vi "Power Supply Loop.vi"(11 "FPGA Ref":T1) -> ()   [LabVIEW 2013]
uses:
  Controls/FPGA_Reference.ctl
  <vilib>/rvi/interface/nirviReadWriteControl/nirviReadWriteControl.xnode
  FPGA Bitfiles/LSDurability_Main.lvbitx
  <vilib>/rvi/errors/niLvFpgaMergeErrorWithErrorCode.vi
  <vilib>/rvi/errors/niLvFpgaAdjustHostInterfaceError.vi
panel:
  in  "Power Supply Cmd (V):":dbl min=0.0 max=20.0 format="%#.2f"
  in  "Closed Loop Voltage":bool
  out "FreezePID":bool
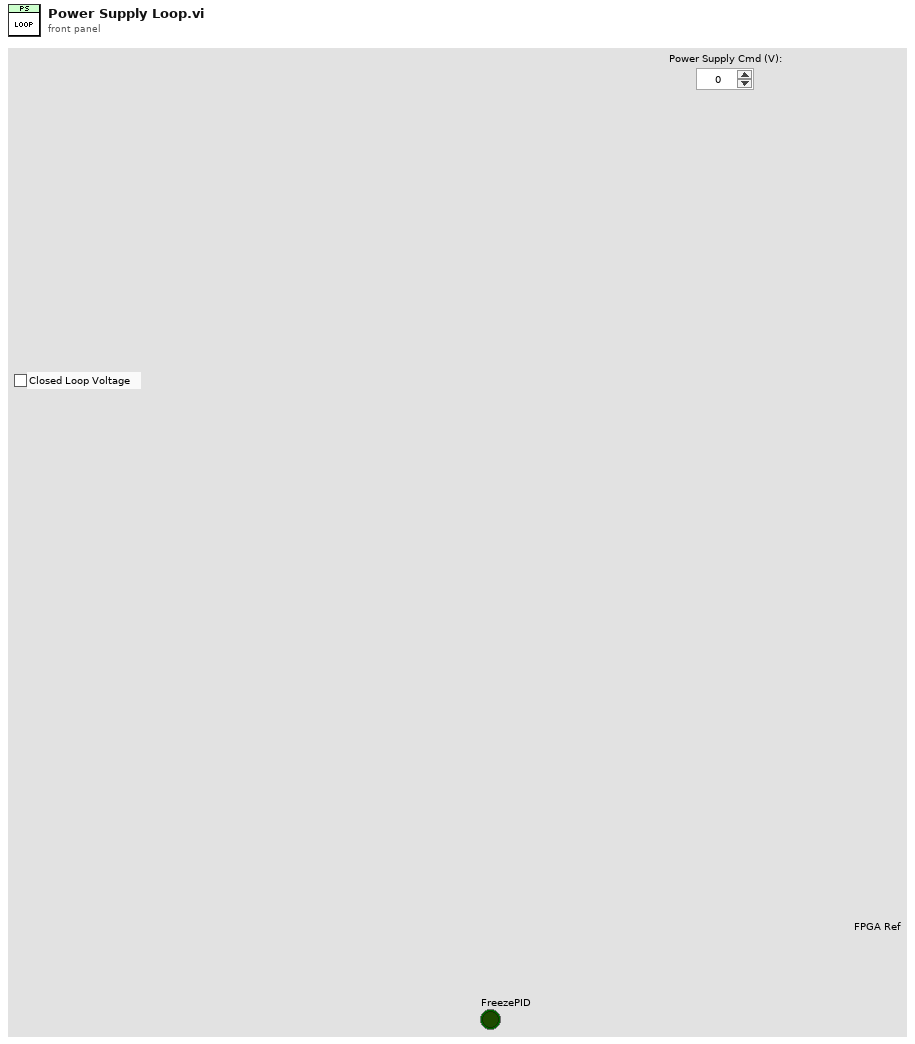
[diagram p1: front panel]
types:
  T1 = typedef "FPGA_Reference.ctl" = refnum<k20>
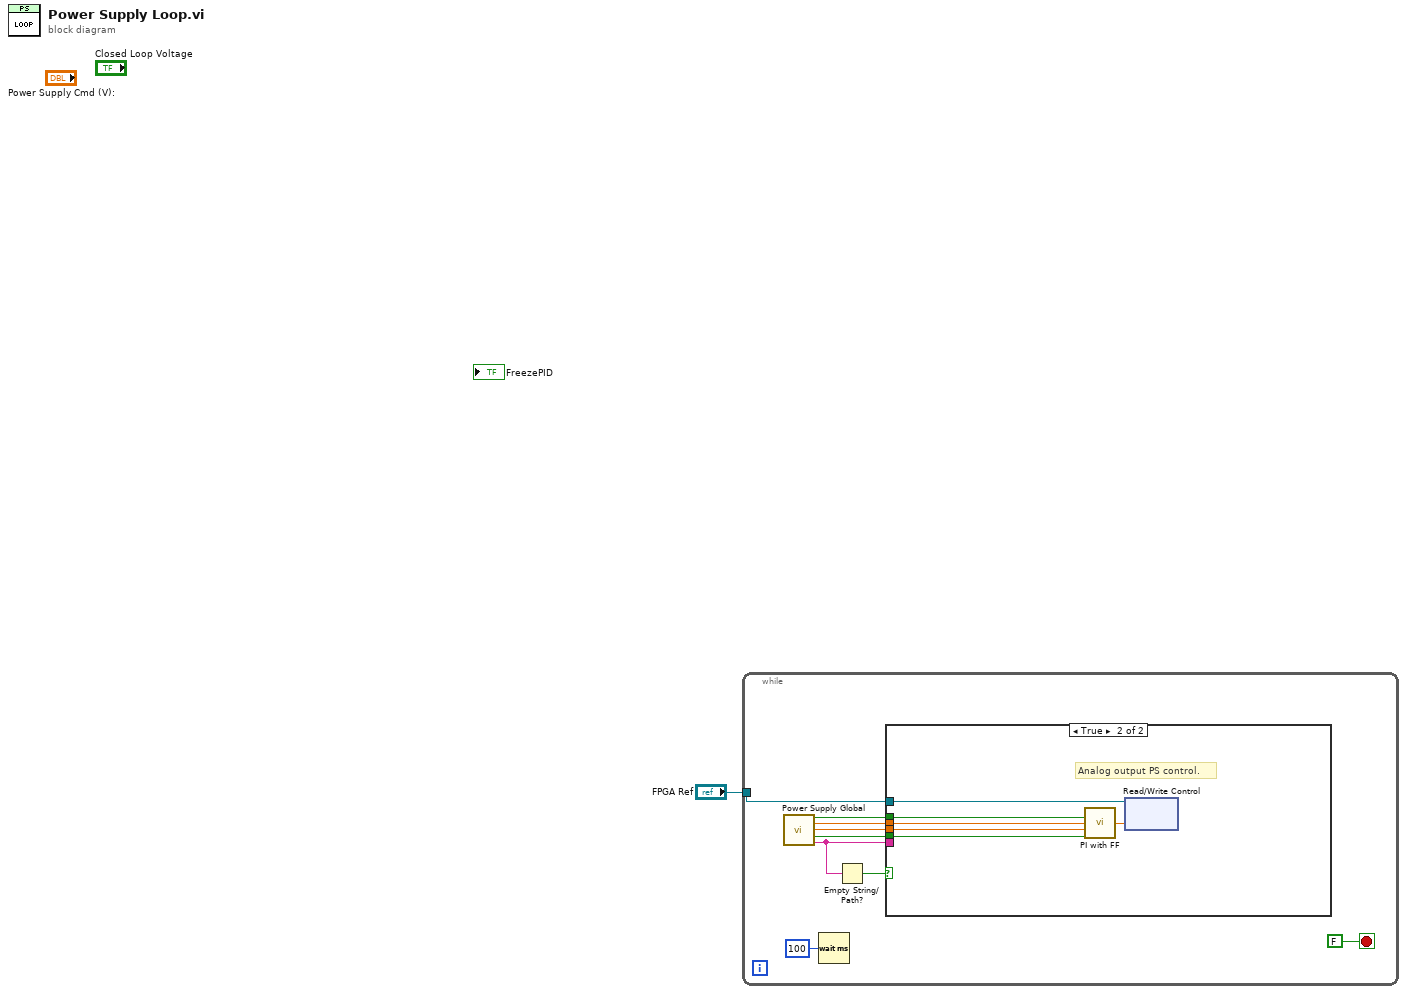
[diagram p0: block diagram]
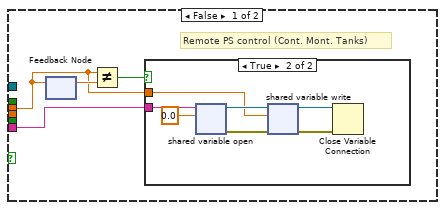
[diagram p2: hidden frame]
diagram:
  n1 = while {
    tunnel: "FPGA Ref" -> [w9]
    stop <- FALSE stop-if-true
    n2 = call "Power Supply Global.vi"() -> ("Closed Loop OUT"=w7:bool, "PS Cmd OUT"=w6:dbl, "PS Voltage OUT"=w5:dbl, "FreezePID OUT"=w4:bool, "VoltCtrlRef OUT"=w2:string)  [unwired: 11 in]
    n3 = Wait (ms)(milliseconds to wait=u32 100) -> ()  [unwired: 1 out]
    n4 = Empty String/Path?(string/path=w2) -> (empty?=w3:bool)
    n5 = case shown="True" w3 {
      tunnel: w9 -> [_ w27]
      tunnel: w7 -> [_ w25]
      tunnel: w6 -> [w11 w24]
      tunnel: w5 -> [_ w23]
      tunnel: w4 -> [_ w22]
      tunnel: w2 -> [w14 _]
      frame False {
        # "Remote PS control (Cont. Mont. Tanks)"
        n6 = feedback-in #1(w11) -> ()
        n7 = feedback #1() -> (w13:dbl)  [unwired: 1 in]
        n8 = Not Equal?(x=w11, y=w13) -> (x != y?=w12:bool)
        n9 = case shown="True" w12 {
          tunnel: w14 -> [_ w16]
          tunnel: w11 -> [_ w15]
          frame False {
          }
          frame True {
            n10 = shared-variable-open(w16, 0.0) -> (w17:refnum<k21>, w20:errorcluster)  [unwired: 2 in]
            n11 = shared-variable-write(w17, w20, w15) -> (w18:refnum<k21>, w19:errorcluster)
            n12 = Close Variable Connection(8:w19, 11:w18) -> ()  [unwired: 1 out]
          }
        }
      }
      frame True {
        # "Analog output PS control."
        n13 = call "PI with FF.vi"("Run PI?"=w25, "SP"=w24, "Actual"=w23, "Freeze Output"=w22) -> ("Output"=w26:dbl)  [unwired: 11 in]
        n14 = xnode "Read/Write Control"("FPGA VI Reference In"=w27, "AO0"=w26) -> ()  [unwired: 1 in, 2 out]
      }
    }
  }
